vi "Standardize Generated API Paths.vi"(8 "error in":errorcluster, 11 "generation data":T1) -> (0 "error out":errorcluster)   [LabVIEW 2024, in "gRPC Client Generation.lvlib"]
uses:
  gRPC Client Generation.lvlib
  Generation Data.ctl
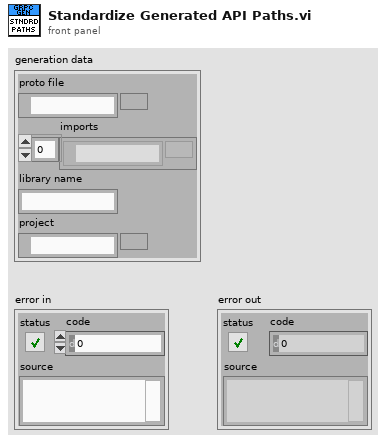
[diagram p1: front panel]
types:
  T1 = typedef "gRPC Client Generation.lvlib/Generation Data.ctl" = cluster{"proto file":path, "imports":path[], "library name":string, "project":path}
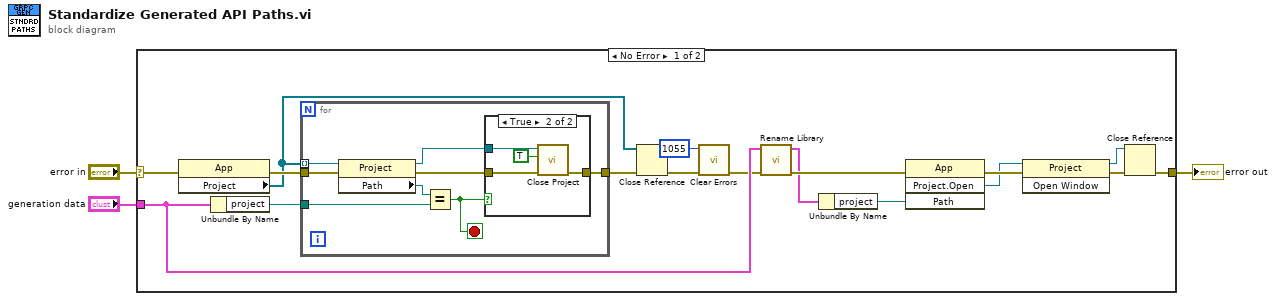
[diagram p0: block diagram]
diagram:
  n1 = case shown="No Error" "error in" {
    selector: "error in" -> [w16 w34]
    tunnel: "generation data" -> [w14 _]
    tunnel: [w8 w34] -> w3
    frame No Error {
      n2 = property class="App"(error in=w16) -> (error out=w19:errorcluster, "Project"=w17:refnum<vi>[])  [unwired: 1 in, 1 out]
      n3 = Unbundle By Name(w14) -> ("project"=w20:path)
      n4 = for {
        tunnel: w17 -> [w28] mode=indexing
        tunnel: w20 -> [w26]
        tunnel: w19 -> [w22]
        tunnel: [w21] -> w18
        stop <- w25 stop-if-true
        n5 = property class="Project"(reference=w28, error in=w22) -> (reference out=w23:refnum<vi>, error out=w24:errorcluster, "Path"=w27:path)
        n6 = Equal?(x=w27, y=w26) -> (x = y?=w25:bool)
        n7 = case shown="True" w25 {
          tunnel: w24 -> [w29 w33]
          tunnel: w23 -> [_ w32]
          tunnel: [w29 w30] -> w21
          frame False {
          }
          frame True {
            n8 = call "Close Project.vi"("error in"=w33, "save"=TRUE, "project ref"=w32) -> ("error out"=w30:errorcluster)  [unwired: 8 in]
          }
        }
      }
      n9 = Close Reference(reference=w17, error in (no error)=w18) -> (error out=w15:errorcluster)
      n10 = call <vilib>:"Clear Errors.vi"("error in (no error)"=w15, "specific error code to clear (0: all)"=1055) -> ("error out"=w5:errorcluster)  [unwired: 4 in, 1 out]
      n11 = call "Rename Library.vi"("generation data"=w14, "error in"=w5) -> ("generation data out"=w7:T1, "error out"=w13:errorcluster)  [unwired: 7 in]
      n12 = Unbundle By Name(w7) -> ("project"=w6:path)
      n13 = invoke class="App" method="Project.Open"(error in=w13, "Path"=w6) -> (error out=w12:errorcluster, "Project:Open"=w11:refnum<vi>)  [unwired: 2 in, 2 out]
      n14 = invoke class="Project" method="Open Window"(reference=w11, error in=w12) -> (reference out=w9:refnum<vi>, error out=w10:errorcluster)  [unwired: 1 in, 1 out]
      n15 = Close Reference(reference=w9, error in (no error)=w10) -> (error out=w8:errorcluster)
    }
    frame Error {
    }
  }
  "error out" <- w3
